vi "Shutdown All Streams.vi"(8 "Error In":errorcluster, 11 "Aircraft ID":u8) -> (0 "error out":errorcluster)   [LabVIEW 2014]
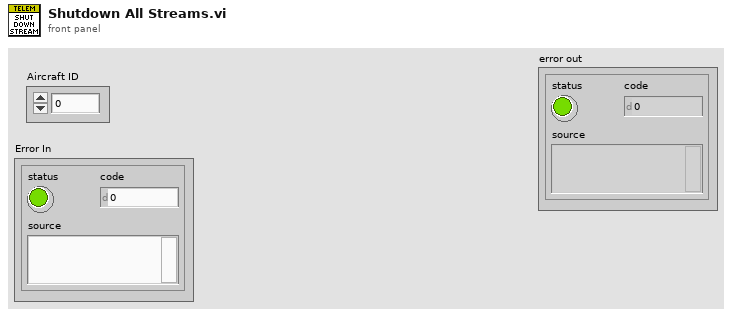
[diagram p1: front panel]
types:
  T1 = enum16{"ALL", "RAW_SENSORS", "EXTENDED_STATUS", "RC_CHANNELS", "RAW_CONTROLLER", "POSITION", "EXTRA1", "EXTRA2", "EXTRA3"}
  T2 = cluster{"req_message_rate":u16, "target_system":u8, "target_component":u8, "req_stream_id":enum16{"ALL", "RAW_SENSORS", "EXTENDED_STATUS", "RC_CHANNELS", "RAW_CONTROLLER", "POSITION", "EXTRA1", "EXTRA2", "EXTRA3"}, "start_stop":bool}
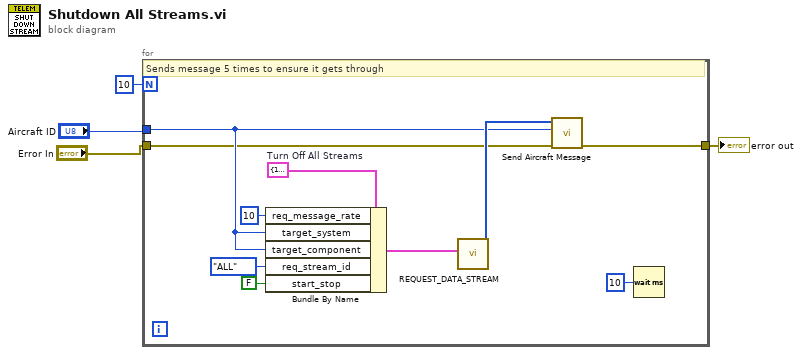
[diagram p0: block diagram]
diagram:
  n1 = for {
    N: 10 -> [_]
    tunnel: "Error In" -> [w5]
    tunnel: [w13] -> w1
    tunnel: "Aircraft ID" -> [w6]
    w11 = T2 {"req_message_rate"=10, "target_system"=1, "target_component"=1, "req_stream_id"=enum."ALL", "start_stop"=FALSE}  # Turn Off All Streams
    # "Sends message 5 times to ensure it gets through"
    n2 = Bundle By Name(cluster=w11, "req_message_rate"=u16 10, "target_system"=w6, "target_component"=w6, "req_stream_id"=T1."ALL", "start_stop"=FALSE) -> (w7:T2)
    n3 = call "REQUEST_DATA_STREAM.vi"("Payload"=w7) -> ("MAVLink MSG"=w12:u8[])  [unwired: 10 in]
    n4 = call "Send Aircraft Message.vi"("error in (no error)"=w5, "Aircraft ID"=w6, "MAVLink Message"=w12) -> ("error out"=w13:errorcluster)  [unwired: 8 in]
    n5 = Wait (ms)(milliseconds to wait=u32 10) -> ()  [unwired: 1 out]
  }
  "error out" <- w1
